vi "Flow Frequencies Global.vi"() -> ()   [LabVIEW 2013]
panel:
  out "Flow Frequencies":fxp<+/-,28,17>[](array[numeric])
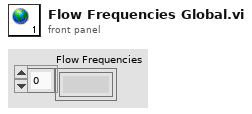
[diagram p1: front panel]
diagram:
